vi "po2sp.vi"(9 "speed":dbl, 10 "P2":cluster{"X":dbl, "Y":dbl}, 11 "P1":cluster{"X":dbl, "Y":dbl}) -> (2 "Vx":dbl, 3 "Vy":dbl)   [LabVIEW 2011]
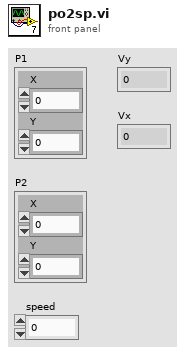
[diagram p1: front panel]
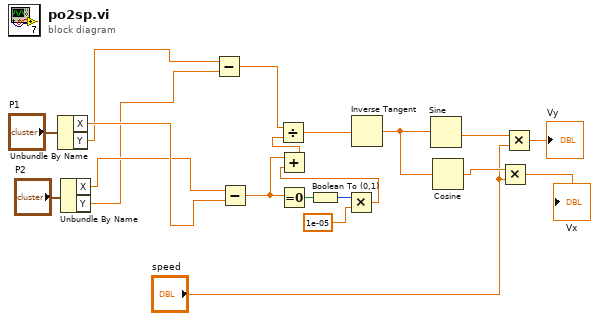
[diagram p0: block diagram]
diagram:
  n1 = Unbundle By Name("P1") -> ("X"=w20:dbl, "Y"=w17:dbl)
  n2 = Unbundle By Name("P2") -> ("X"=w19:dbl, "Y"=w18:dbl)
  n3 = Subtract(x=w17, y=w18) -> (x-y=w14:dbl)
  n4 = Subtract(x=w19, y=w20) -> (x-y=w2:dbl)
  n5 = Equal To 0?(x=w2) -> (x = 0?=w6:bool)
  n6 = Boolean To (0,1)(Boolean=w6) -> (0, 1=w5:i16)
  n7 = Multiply(x=w5, y=1e-05) -> (x*y=w3:dbl)
  n8 = Add(x=w2, y=w3) -> (x+y=w1:dbl)
  n9 = Divide(x=w14, y=w1) -> (x/y=w13:dbl)
  n10 = Inverse Tangent(1:w13) -> (0:w12:dbl)
  n11 = Sine(x=w12) -> (sin(x)=w10:dbl)
  n12 = Cosine(x=w12) -> (cos(x)=w11:dbl)
  n13 = Multiply(x=w11, y="speed") -> (x*y=→"Vx":dbl)
  n14 = Multiply(x=w10, y="speed") -> (x*y=→"Vy":dbl)
